vi "Set TDMS logfile.vi"(7 "TDMS Module Alias":string, 8 "log name":string, 9 "Log Directory":string, 10 "Config File Save Path":path, 11 "Config File Path":path) -> (0 "error out":errorcluster)   [LabVIEW 2014]
doc: "Update the log file a TDMS module will write to"
uses:
  <vilib>/NI/DCAF/Modules/TDMS Datalogger/configuration/TDMS datalogger configuration.lvclass
  <vilib>/NI/DCAF/Modules/TDMS Datalogger/configuration/TDMS datalogger configuration.lvclass/TDMS datalogger configuration.ctl
  <vilib>/NI/Configuration Framework/tree serializer/NISE_CEF_TreeSerializer.lvlib
  <vilib>/NI/DCAF/Tag Editor Core/Framework Configuration Classes/class cache/PL_class cache.lvlib
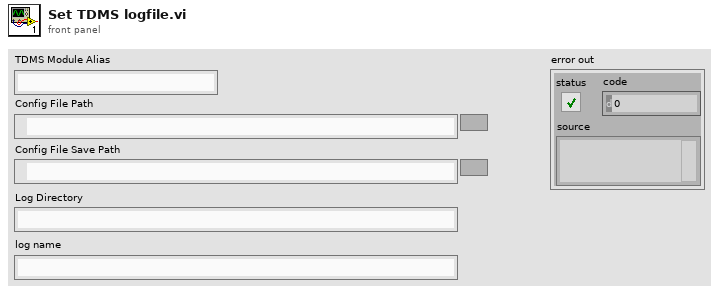
[diagram p1: front panel]
types:
  T1 = typedef "PL_class cache.lvlib/cache definition.ctl" = cluster{"configuration":T2, "class cache data":T3}
  T2 = typedef "PL_class cache.lvlib/cache search configuration.ctl" = cluster{"Search Paths":path[], "Folders to Exclude":string[], "full class list":path[]}
  T3 = typedef "PL_class cache.lvlib/cached class information.ctl" = cluster{"targets":T4[], "engines":T5[], "modules":T5[], "ignored class list":path[]}
  T4 = typedef "PL_class cache.lvlib/target class metadata.ctl" = cluster{"file name":string, "fully qualified name":string, "menu display name":string, "configuration class name":string}
  T5 = typedef "PL_class cache.lvlib/class metadata.ctl" = cluster{"file name":string, "fully qualified name":string, "menu display name":string, "configuration class":string, "category":string, "instances allowed":i32, "supported targets":T6[]}
  T6 = typedef "TBM configuration.lvclass/Target Types.ctl" = enum16{"Windows", "Mac", "Linux", "Linux RT ARM", "VxWorks", "Pharlap", "Other", "Linux RT x64"}
  T7 = typedef "NISE_CEF_TreeSerializer.lvlib/base file format.ctl" = cluster{"version":string, "data":string}
  T8 = typedef "NISE_CEF_TreeSerializer.lvlib/flat hierarchy.ctl" = cluster{"hierarchy structure":T9, "instance data":T11[]}
  T9 = typedef "NISE_CEF_TreeSerializer.lvlib/full hierarchy.ctl" = cluster{"root":string, "hierarchy":T10[]}
  T10 = typedef "NISE_CEF_TreeSerializer.lvlib/hierarchy element.ctl" = cluster{"current node":string, "children":string[]}
  T11 = typedef "NISE_CEF_TreeSerializer.lvlib/instance data.ctl" = cluster{"ID":string, "Alias":string, "class":string, "version":string, "data":string}
  T12 = typedef "NISE_CEF_TreeSerializer.lvlib/memory hierarchy.ctl" = cluster{"hierarchy structure":T9, "instance data":refnum<class "NISE_CEF_serializable configuration.lvclass">[]}
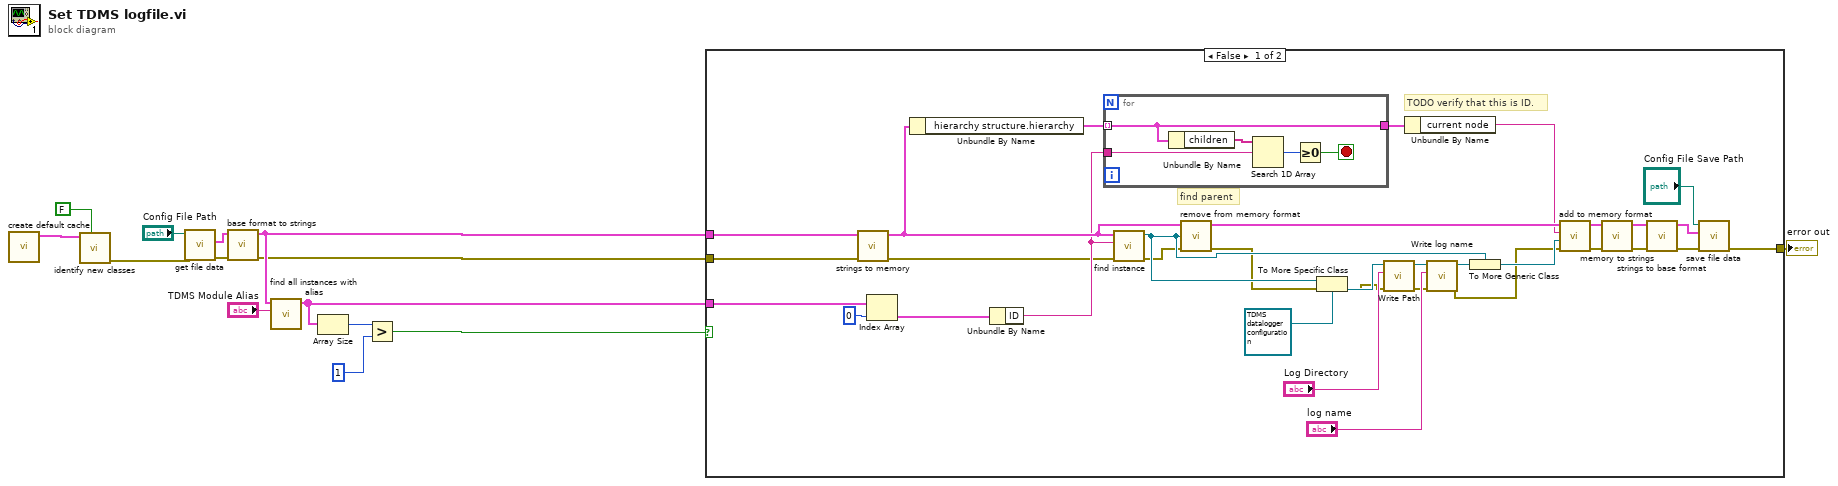
[diagram p0: block diagram]
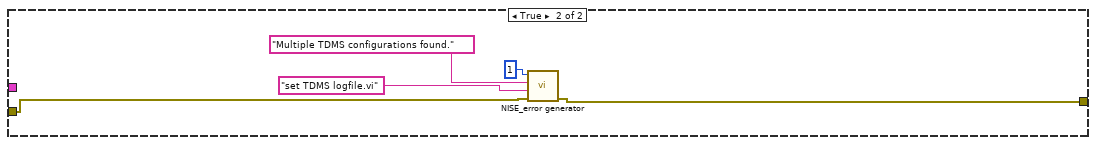
[diagram p2: hidden frame]
diagram:
  n1 = call <vilib>:"create default cache.vi"() -> ("cache"=w3:T1)  [unwired: 11 in]
  n2 = call <vilib>:"identify new classes.vi"("existing progress bar?"=FALSE, "cache in"=w3) -> ("error out"=w2:errorcluster)  [unwired: 8 in, 1 out]
  n3 = call <vilib>:"get file data.vi"("error in"=w2, "Path"="Config File Path") -> ("error out"=w14:errorcluster, "format"=w13:T7)  [unwired: 8 in]
  n4 = call <vilib>:"base format to strings.vi"("error in"=w14, "format"=w13) -> ("error out"=w8:errorcluster, "data"=w10:T8)  [unwired: 8 in]
  n5 = call <vilib>:"find all instances with alias.vi"("Alias"="TDMS Module Alias", "flat hierarchy"=w10) -> ("instance data"=w7:T11[])  [unwired: 9 in]
  n6 = Array Size(array=w7) -> (size(s)=w6:i32)
  n7 = Greater?(x=w6, y=1) -> (0:w4:bool)
  n8 = case shown="False" w4 {
    tunnel: w10 -> [w43 _]
    tunnel: [w22 w53] -> w9
    tunnel: w8 -> [w20 w54]
    tunnel: w7 -> [w15 _]
    frame False {
      # "TODO verify that this is ID."
      # "find parent"
      n9 = call <vilib>:"strings to memory.vi"("error in"=w20, "1.0.0"=w43) -> ("error out"=w19:errorcluster, "memory hierarchy"=w29:T12)  [unwired: 8 in]
      n10 = Index Array(array=w15, index=0) -> (element=w44:T11)
      n11 = Unbundle By Name(w29) -> ("hierarchy structure.hierarchy"=w28:T10[])
      n12 = Unbundle By Name(w44) -> ("ID"=w27:string)
      n13 = for {
        tunnel: w28 -> [w50] mode=indexing
        tunnel: w27 -> [w51]
        tunnel: [w50] -> w26
        stop <- w48 stop-if-true
        n14 = Unbundle By Name(w50) -> ("children"=w52:string[])
        n15 = Search 1D Array(1D array=w52, element=w51) -> (index of element=w49:i32)  [unwired: 1 in]
        n16 = Greater Or Equal To 0?(x=w49) -> (x >= 0?=w48:bool)
      }
      n17 = call <vilib>:"find instance.vi"("error in"=w19, "ID"=w27, "memory hierarchy"=w29) -> ("error out"=w17:errorcluster, "configuration"=w31:refnum<class "NISE_CEF_serializable configuration.lvclass">)  [unwired: 7 in]
      n18 = call <vilib>:"remove from memory format.vi"("error in"=w17, "NISE_CEF_serializable configuration in"=w31, "memory hierarchy in"=w29) -> ("error out"=w16:errorcluster, "memory hierarchy out"=w30:T12)  [unwired: 7 in]
      n19 = To More Specific Class(target class=refnum<class "TDMS datalogger configuration.lvclass"> refnum ("TDMS datalogger configuration"), reference=w31, error in=w16) -> (specific class reference=w42:refnum<class "TDMS datalogger configuration.lvclass">, error out=w38:errorcluster)
      n20 = call <vilib>:"Write Path.vi"("error in (no error)"=w38, "Log Directory"="Log Directory", "TDMS datalogger configuration in"=w42) -> ("error out"=w37:errorcluster, "TDMS datalogger configuration out"=w40:refnum<class "TDMS datalogger configuration.lvclass">)  [unwired: 7 in]
      n21 = Unbundle By Name(w26) -> ("current node"=w25:string)
      n22 = call <vilib>:"Write log name.vi"("error in (no error)"=w37, "log name"="log name", "TDMS datalogger configuration in"=w40) -> ("error out"=w18:errorcluster, "TDMS datalogger configuration out"=w36:refnum<class "TDMS datalogger configuration.lvclass">)  [unwired: 7 in]
      n23 = To More Generic Class(target class=w31, reference=w36) -> (generic class reference=w32:refnum<class "NISE_CEF_serializable configuration.lvclass">)
      n24 = call <vilib>:"add to memory format.vi"("error in"=w18, "NISE_CEF_serializable configuration in"=w32, "parent ID"=w25, "memory hierarchy in"=w30) -> ("error out"=w33:errorcluster, "memory hierarchy out"=w34:T12)  [unwired: 6 in]
      n25 = call <vilib>:"memory to strings.vi"("error in"=w33, "memory hierarchy"=w34) -> ("error out"=w23:errorcluster, "1.0.0"=w24:T8)  [unwired: 8 in]
      n26 = call <vilib>:"strings to base format.vi"("error in"=w23, "1.0.0"=w24) -> ("error out"=w47:errorcluster, "format"=w46:T7)  [unwired: 8 in]
      n27 = call <vilib>:"save file data.vi"("error in"=w47, "format"=w46, "Path"="Config File Save Path") -> ("error out"=w22:errorcluster)  [unwired: 8 in]
    }
    frame True {
      n28 = call <vilib>:"NISE_error generator.vi"("error in"=w54, "source"="set TDMS logfile.vi", "append error message"="Multiple TDMS configurations found.", "error code (0)"=1) -> ("error out"=w53:errorcluster)  [unwired: 5 in]
    }
  }
  "error out" <- w9
